vi "TestExec.Set Single Test Repeat.vi"(7 "Module Q Name":string, 8 "error in":errorcluster, 10 "Sec Delay":dbl=1.0, 11 "Q In":refnum<queue>) -> (0 "error out":errorcluster, 3 "Q Out":refnum<queue>)   [LabVIEW 2018]
uses:
  <vilib>/KATE/Queues/Q.Element.ctl
  <vilib>/KATE/Queues/Queue Utils.lvlib
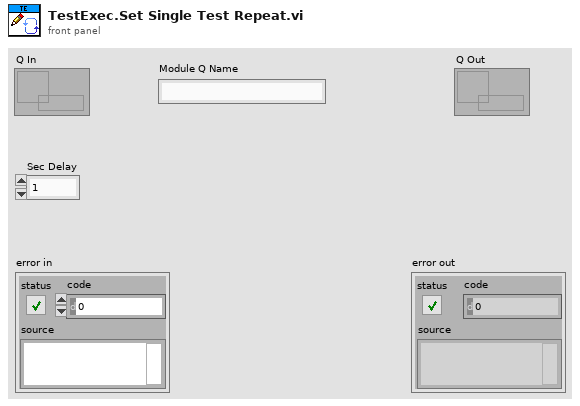
[diagram p1: front panel]
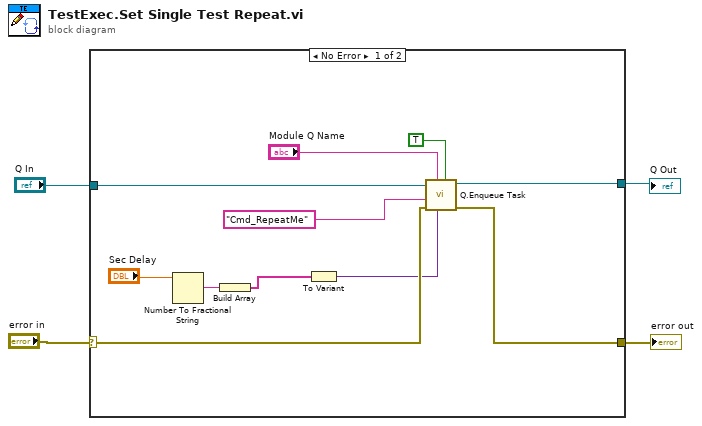
[diagram p0: block diagram]
diagram:
  n1 = case shown="No Error" "error in" {
    selector: "error in" -> [w13 w17]
    tunnel: [w14 w17] -> w3
    tunnel: [w9 w16] -> w2
    tunnel: "Q In" -> [w8 w16]
    frame No Error {
      n2 = Number To Fractional String(number="Sec Delay") -> (F-format string=w5:string)  [unwired: 3 in]
      n3 = Build Array(w5) -> (w6:string[])
      n4 = To Variant(anything=w6) -> (Variant=w12:variant)
      n5 = call <vilib>:"Q.Enqueue Task.vi"("Top of Q"=TRUE, "Data1"=w12, "Q Name"="Module Q Name", "Error In"=w13, "Task Name"="Cmd_RepeatMe" ("Cmd"), "Q In"=w8) -> ("error out"=w14:errorcluster, "Q Out"=w9:refnum<queue>)  [unwired: 4 in]
    }
    frame Error {
    }
  }
  "error out" <- w3
  "Q Out" <- w2
